vi "timeslotsSave.vi"(2 "error in":errorcluster) -> (0 "error out":errorcluster, 1 "array of clusters":T1(array[cluster]))   [LabVIEW 2017]
panel:
  out "size(s)":i32[](array[numeric])
  in  "Array 12":string[](array[string])
  out "Array 11":string[](array[string])
  in  "Array 10":string[](array[string])
  out "Array 9":string[](array[string])
  in  "Array 8":u32[](array[numeric])
  out "Array 7":u32[](array[numeric])
  in  "Array 6":u32[](array[numeric])
  out "Array 5":u32[](array[numeric])
  in  "Array 4":i32[](array[numeric])
  out "Array 3":i32[](array[numeric])
  in  "Array 2":i32[](array[numeric])
  out "array":string[][](array[string])
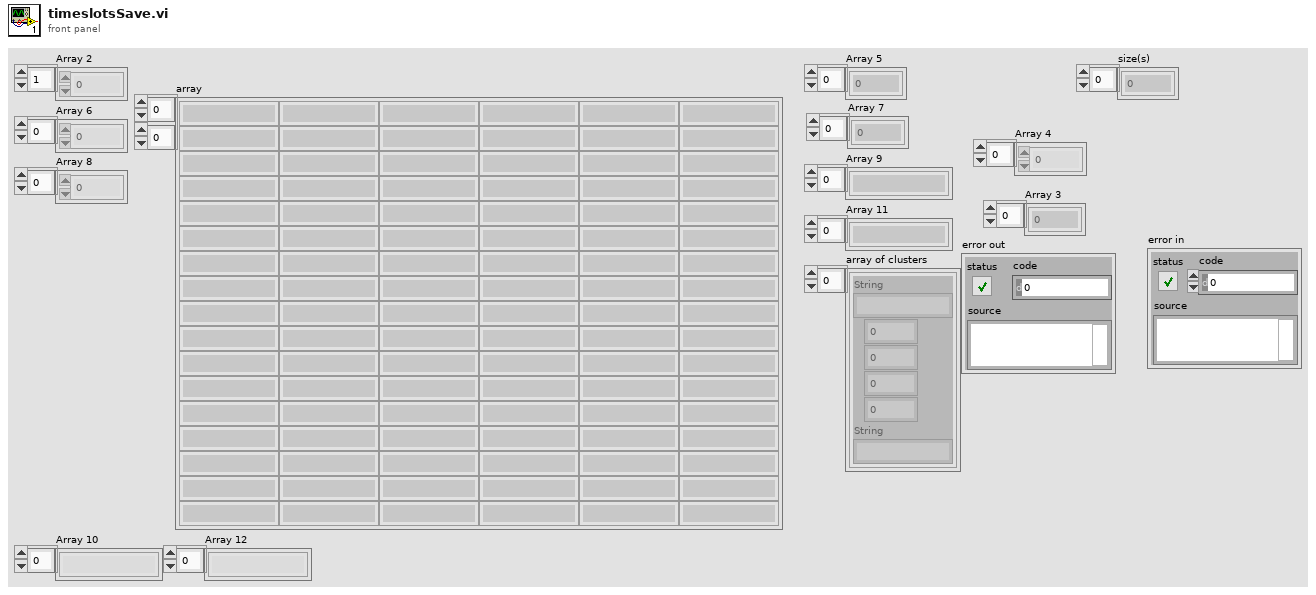
[diagram p1: front panel]
types:
  T1 = cluster{"String":string, i32, i32, u32, u32, "String":string}[]
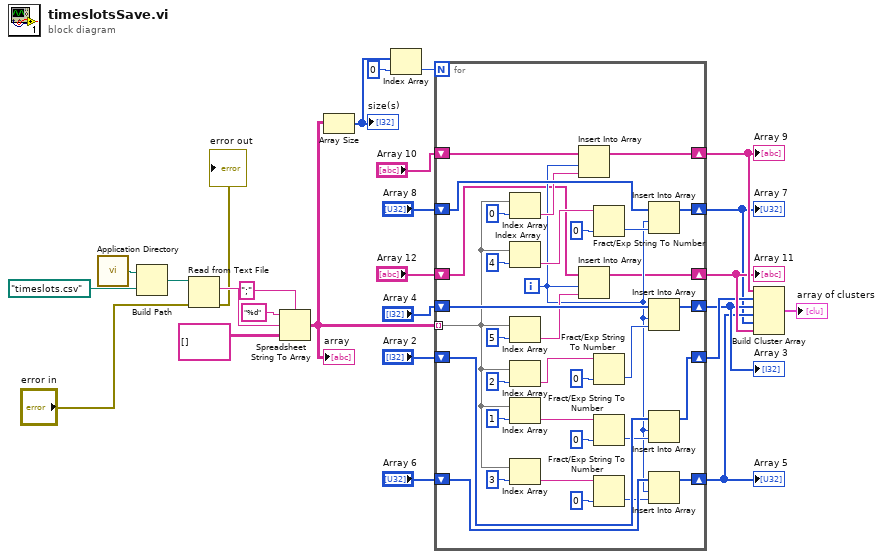
[diagram p0: block diagram]
diagram:
  n1 = call <vilib>:"Application Directory.vi"() -> ("Application Directory"=w21:path)
  n2 = Build Path(base path=w21, name or relative path=path "timeslots.csv" ("default name")) -> (appended path=w22:path)
  n3 = Read from Text File(file (use dialog)=w22, error in="error in") -> (text=w25:string, error out=→"error out":errorcluster)  [unwired: 2 in, 2 out]
  n4 = Spreadsheet String To Array(delimiter (Tab)=";", format string="%d", spreadsheet string=w25, array type (2D Dbl)=string[][] [] ("Array")) -> (array=w13:string[][])
  "array" <- w13
  n5 = Array Size(array=w13) -> (size(s)=w12:i32[])
  "size(s)" <- w12
  n6 = Index Array(array=w12, index=0) -> (element=w10:i32)
  n7 = for {
    N: w10 -> [_]
    tunnel: w13 -> [w29] mode=indexing
    shift-right: [w56] -> w7
    shift-left: "Array 2" -> [w57]
    shift-right: [w49] -> w6
    shift-left: "Array 4" -> [w50]
    shift-right: [w48] -> w5
    shift-left: "Array 6" -> [w47]
    shift-right: [w37] -> w4
    shift-left: "Array 8" -> [w38]
    shift-right: [w35] -> w9
    shift-left: "Array 10" -> [w34]
    shift-right: [w31] -> w8
    shift-left: "Array 12" -> [w30]
    i -> [w32]
    n8 = Index Array(array=w29, index=0) -> (element=w36:string)
    n9 = Index Array(array=w29, index=4) -> (element=w43:string)
    n10 = Index Array(array=w29, index=5) -> (element=w33:string)
    n11 = Index Array(array=w29, index=2) -> (element=w53:string)
    n12 = Index Array(array=w29, index=1) -> (element=w59:string)
    n13 = Index Array(array=w29, index=3) -> (element=w44:string)
    n14 = Insert Into Array(array=w34, index=w32, new element=w36) -> (w35:string[])
    n15 = Insert Into Array(array=w30, index=w32, new element=w33) -> (w31:string[])
    n16 = Fract/Exp String To Number(string=w43, default (0 dbl)=u32 0 ("default (0 DBL)")) -> (number=w39:u32)  [unwired: 2 in, 1 out]
    n17 = Fract/Exp String To Number(string=w53, default (0 dbl)=u32 0 ("default (0 DBL)")) -> (number=w51:u32)  [unwired: 2 in, 1 out]
    n18 = Fract/Exp String To Number(string=w59, default (0 dbl)=u32 0 ("default (0 DBL)")) -> (number=w55:u32)  [unwired: 2 in, 1 out]
    n19 = Fract/Exp String To Number(string=w44, default (0 dbl)=u32 0 ("default (0 DBL)")) -> (number=w40:u32)  [unwired: 2 in, 1 out]
    n20 = Insert Into Array(array=w38, index=w32, new element=w39) -> (w37:u32[])
    n21 = Insert Into Array(array=w50, index=w32, new element=w51) -> (w49:i32[])
    n22 = Insert Into Array(array=w57, index=w32, new element=w55) -> (w56:i32[])
    n23 = Insert Into Array(array=w47, index=w32, new element=w40) -> (w48:u32[])
  }
  "Array 3" <- w6
  "Array 5" <- w5
  "Array 7" <- w4
  "Array 9" <- w9
  "Array 11" <- w8
  n24 = Build Cluster Array(w9, w7, w6, w5, w4, w8) -> (→"array of clusters":T1)
